vi "Query Parameter XML File - 664.vi"(0 "Path in":path=path "C:/work/SE/Opportunities/2012/Pilatus/201210/TestXMLs/Receiver.xml", 5 "664 Device Without Parameters":T1, 11 "error in (no error)":errorcluster) -> (6 "664 Device With Parameters Out":T1, 15 "error out":errorcluster)   [LabVIEW 2013, in "AIT 664 Custom Device.lvlib"]
doc: "Run through all Messages defined in the Simulyzer configuration. If any matches in the parameters\nconfiguration, pull them in, else, ignore.\n\nThis will leave parameter definitions without corresponding messages out of the import."
uses:
  AIT 664 Custom Device.lvlib
  Controls/664 - XML Device Description.ctl
  Controls/664 - XML End System Description.ctl
  Controls/664 - XML Output VL.ctl
  Controls/664 - XML Tx Message Port.ctl
  Controls/664 - Sampling Type.ctl
  Controls/664 -Param.ctl
  Controls/664 - XML Input VL.ctl
  Controls/664 - XML Rx Message Port.ctl
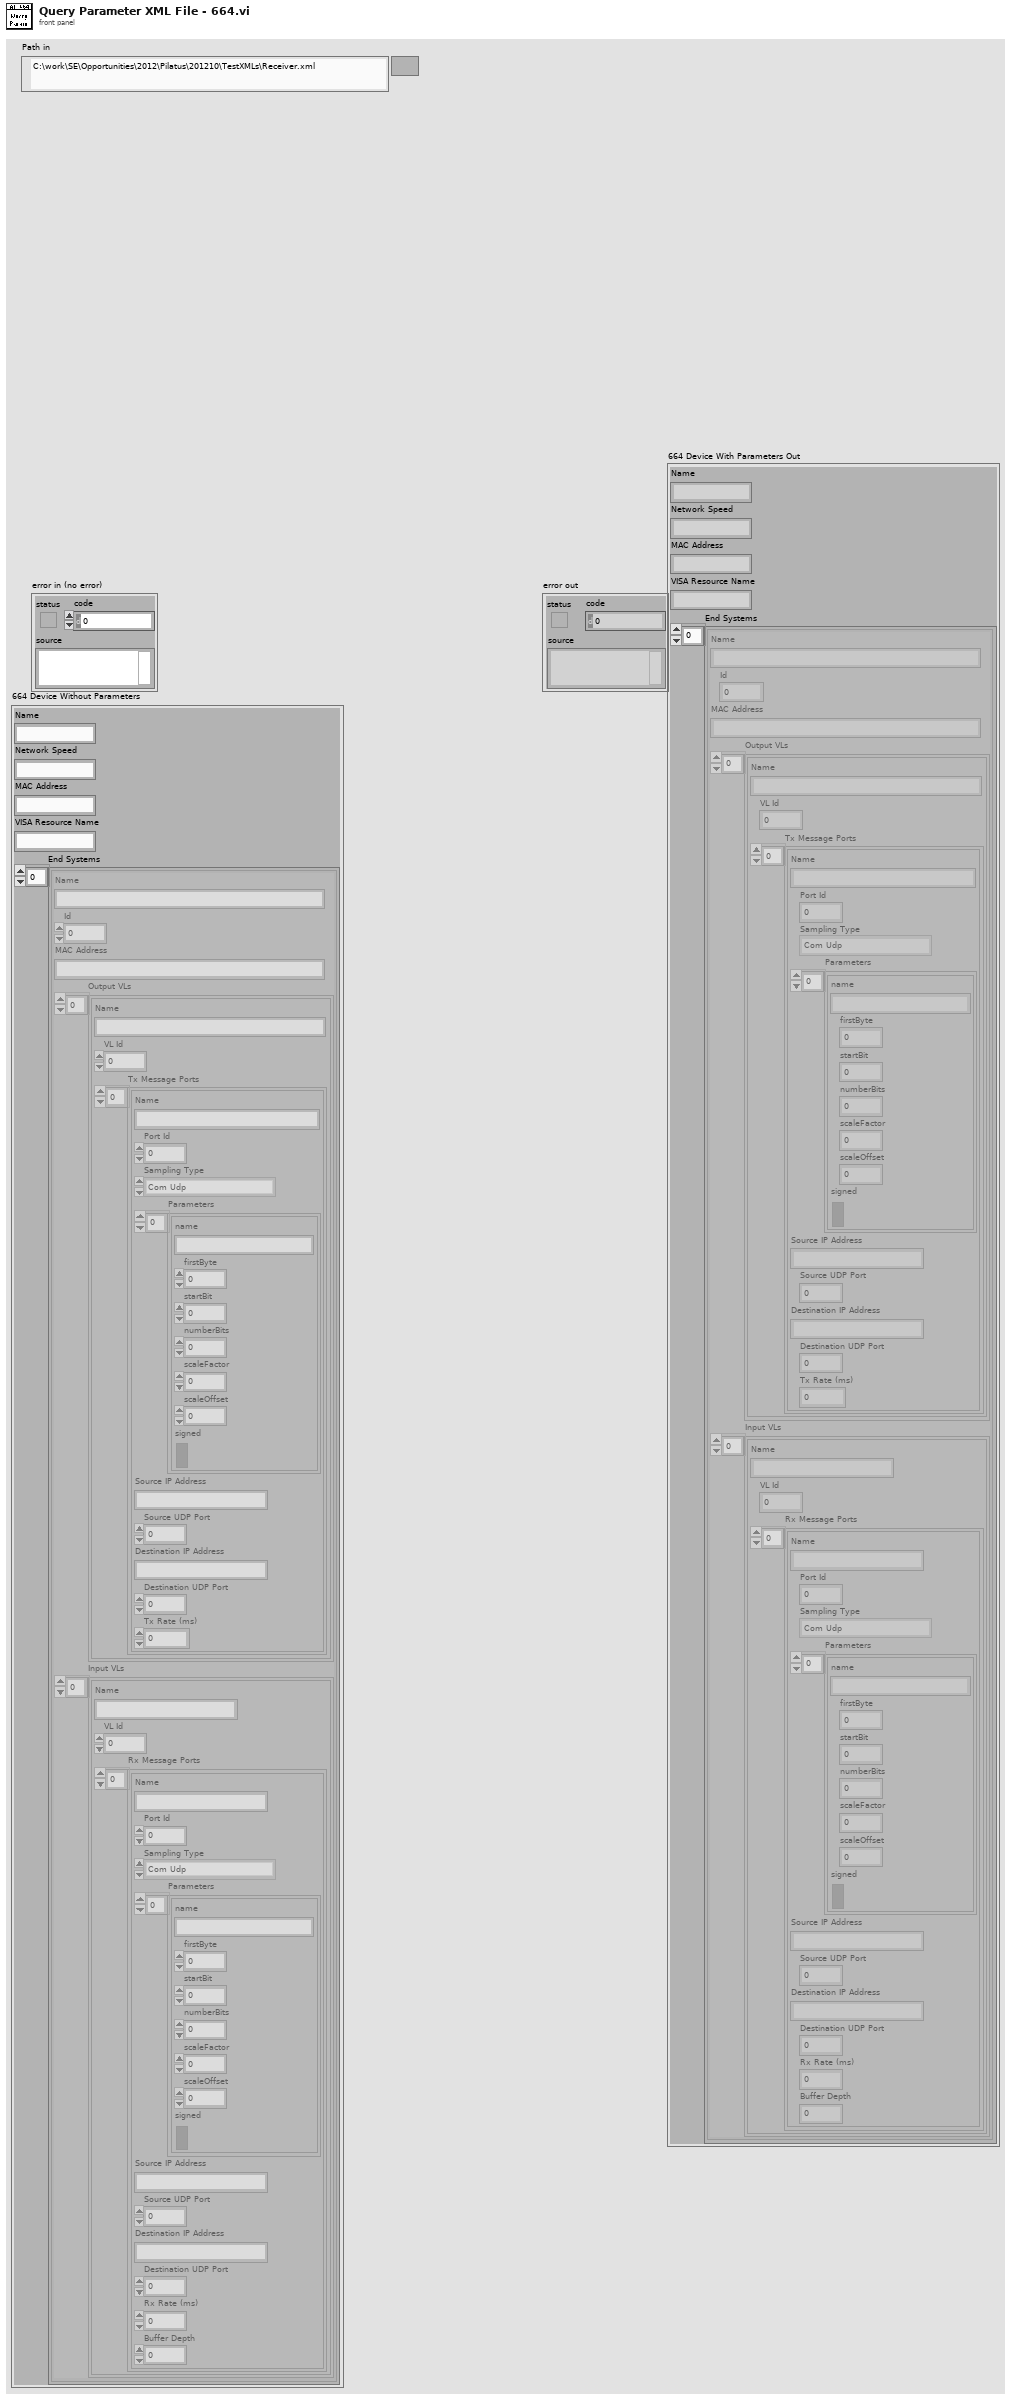
[diagram p1: front panel]
types:
  T1 = typedef "AIT 664 Custom Device.lvlib/664 - XML Device Description.ctl" = cluster{"Name":string, "Network Speed":string, "MAC Address":string, "VISA Resource Name":string, "End Systems":T2[]}
  T2 = typedef "AIT 664 Custom Device.lvlib/664 - XML End System Description.ctl" = cluster{"Name":string, "Id":u32, "MAC Address":string, "Output VLs":T3[], "Input VLs":T7[]}
  T3 = typedef "AIT 664 Custom Device.lvlib/664 - XML Output VL.ctl" = cluster{"Name":string, "VL Id":u32, "Tx Message Ports":T4[]}
  T4 = typedef "AIT 664 Custom Device.lvlib/664 - XML Tx Message Port.ctl" = cluster{"Name":string, "Port Id":u32, "Sampling Type":T5, "Parameters":T6[], "Source IP Address":string, "Source UDP Port":u32, "Destination IP Address":string, "Destination UDP Port":u32, "Tx Rate (ms)":u32}
  T5 = typedef "AIT 664 Custom Device.lvlib/664 - Sampling Type.ctl" = enum16{"Com Udp", "Com Udp Queuing", "Sap Udp", "Sap Ip", "Sap Mac", "Unknown"}
  T6 = typedef "AIT 664 Custom Device.lvlib/664 -Param.ctl" = cluster{"name":string, "firstByte":i32, "startBit":i32, "numberBits":i32, "scaleFactor":dbl, "scaleOffset":dbl, "signed":bool}
  T7 = typedef "AIT 664 Custom Device.lvlib/664 - XML Input VL.ctl" = cluster{"Name":string, "VL Id":u32, "Rx Message Ports":T8[]}
  T8 = typedef "AIT 664 Custom Device.lvlib/664 - XML Rx Message Port.ctl" = cluster{"Name":string, "Port Id":u32, "Sampling Type":T5, "Parameters":T6[], "Source IP Address":string, "Source UDP Port":u32, "Destination IP Address":string, "Destination UDP Port":u32, "Rx Rate (ms)":u32, "Buffer Depth":u32}
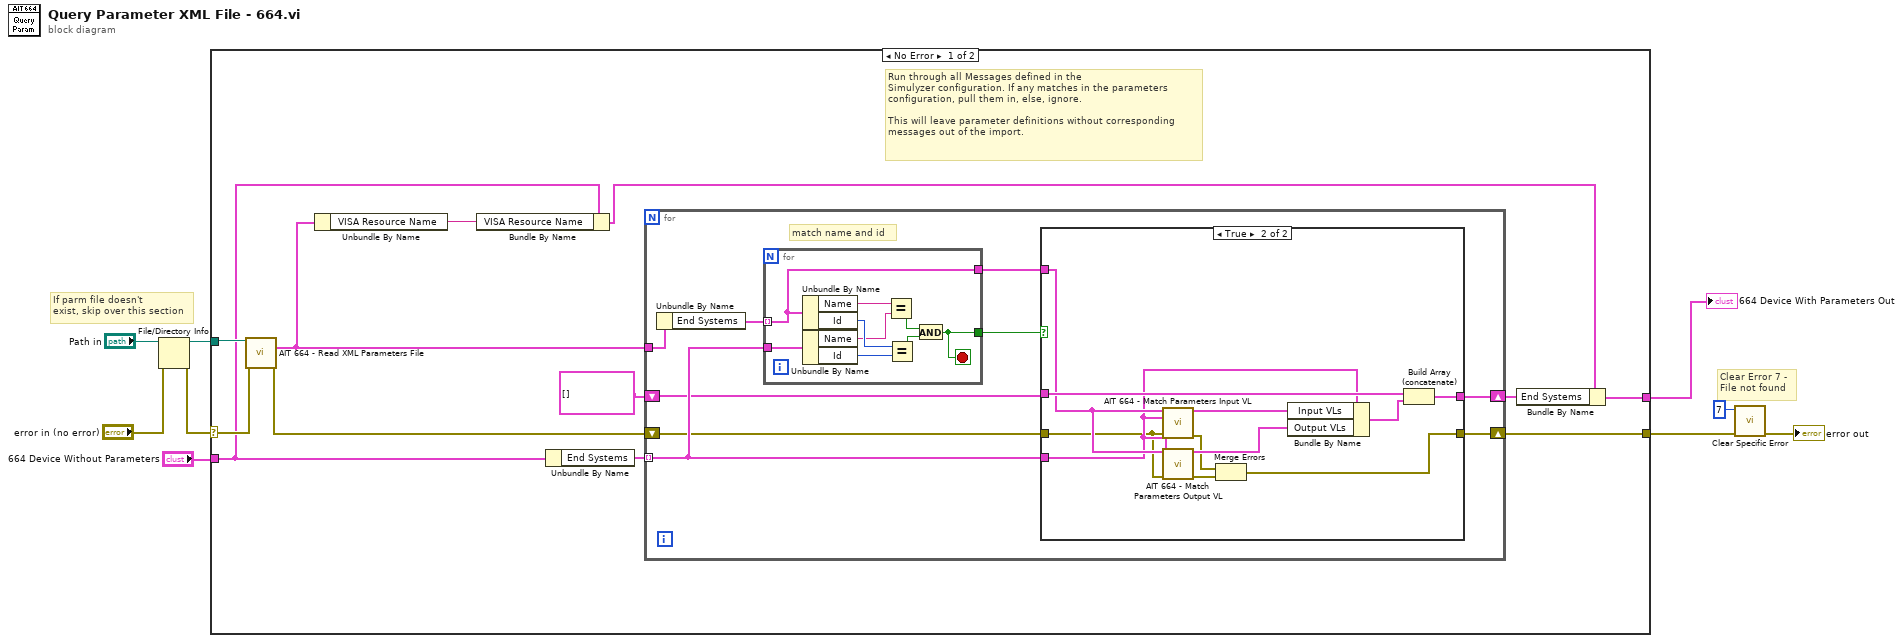
[diagram p0: block diagram]
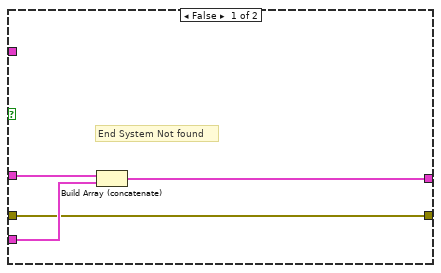
[diagram p2: hidden frame]
diagram:
  # "If parm file doesn't\nexist, skip over this section"
  # "Clear Error 7 - \nFile not found"
  n1 = File/Directory Info(path="Path in", error in="error in (no error)") -> (path out=w9:path, error out=w5:errorcluster)  [unwired: 5 out]
  n2 = case shown="No Error" w5 {
    selector: w5 -> [w20 w55]
    tunnel: [w19 w56] -> w1
    tunnel: w9 -> [w21 _]
    tunnel: [w14 w55] -> w7
    tunnel: "664 Device Without Parameters" -> [w13 w56]
    frame No Error {
      # "Run through all Messages defined in the\nSimulyzer configuration. If any matches in the parameters\nconfiguration, pull them in, else, ignore.\n\nThis will leave parameter definitions without corresponding\nmessages out of the import."
      n3 = call "AIT 664 - Read XML Parameters File.vi"("File Path"=w21, "error in (no error)"=w20) -> ("664 Device Out"=w11:T1, "error out"=w18:errorcluster)  [unwired: 12 in]
      n4 = Unbundle By Name(w11) -> ("VISA Resource Name"=w10:string)
      n5 = Bundle By Name(cluster=w13, "VISA Resource Name"=w10) -> (w12:T1)
      n6 = Unbundle By Name(w13) -> ("End Systems"=w17:T2[])
      n7 = for {
        tunnel: w11 -> [w29]
        shift-right: [w22] -> w14
        shift-left: w18 -> [w23]
        tunnel: w17 -> [w26] mode=indexing
        shift-right: [w25] -> w16
        shift-left: T2[] [] -> [w24]
        # "match name and id"
        n8 = Unbundle By Name(w29) -> ("End Systems"=w30:T2[])
        n9 = for {
          tunnel: w30 -> [w53] mode=indexing
          tunnel: w26 -> [w54]
          tunnel: [w53] -> w27
          tunnel: [w46] -> w28
          stop <- w46 stop-if-true
          n10 = Unbundle By Name(w53) -> ("Name"=w50:string, "Id"=w51:u32)
          n11 = Unbundle By Name(w54) -> ("Name"=w49:string, "Id"=w52:u32)
          n12 = Equal?(x=w50, y=w49) -> (x = y?=w47:bool)
          n13 = Equal?(x=w51, y=w52) -> (x = y?=w48:bool)
          n14 = And(x=w47, y=w48) -> (x .and. y?=w46:bool)
        }
        n15 = case shown="True" w28 {
          tunnel: w27 -> [_ w41]
          tunnel: w26 -> [w34 w40]
          tunnel: [w32 w43] -> w25
          tunnel: w24 -> [w33 w42]
          tunnel: w23 -> [w31 w38]
          tunnel: [w31 w35] -> w22
          frame False {
            # "End System Not found"
            n16 = Build Array (concatenate)(w33, w34) -> (w32:T2[])
          }
          frame True {
            n17 = call "AIT 664 - Match Parameters Input VL.vi"("664 End System Parameter File"=w41, "664 End System Configuration File"=w40, "error in"=w38) -> ("Input VLs out"=w45:T7[], "error out"=w36:errorcluster)  [unwired: 11 in]
            n18 = call "AIT 664 - Match Parameters Output VL.vi"("664 End System Parameter File"=w41, "664 End System Configuration File"=w40, "error in"=w38) -> ("Outyput VLs out"=w39:T3[], "error out"=w37:errorcluster)  [unwired: 11 in]
            n19 = Merge Errors(w36, w37) -> (w35:errorcluster)
            n20 = Bundle By Name(cluster=w40, "Input VLs"=w45, "Output VLs"=w39) -> (w44:T2)
            n21 = Build Array (concatenate)(w42, w44) -> (w43:T2[])
          }
        }
      }
      n22 = Bundle By Name(cluster=w12, "End Systems"=w16) -> (w19:T1)
    }
    frame Error {
    }
  }
  "664 Device With Parameters Out" <- w1
  n23 = call "Clear Specific Error.vi"("error in (no error)"=w7, "code"=7) -> ("error out"=→"error out":errorcluster)  [unwired: 8 in, 1 out]
